vi "Run Bfr Rx - Prepend Size.vi"(7 "Data Size":i32, 8 "error in (no error)":errorcluster, 11 "Data Buffer in":u64 format="%016x") -> (0 "error out":errorcluster, 3 "Data Buffer out":u64 format="%016x")   [LabVIEW 2016, in "UDP-Custom-Device Engine.lvlib"]
uses:
  UDP-Custom-Device Engine.lvlib
  <vilib>/NI Veristand/VeriStand Data/Library/Pointer Operations/Pointer.Write (I32).vi
  <vilib>/NI Veristand/VeriStand Data/Library/VeriStand Data.lvlib
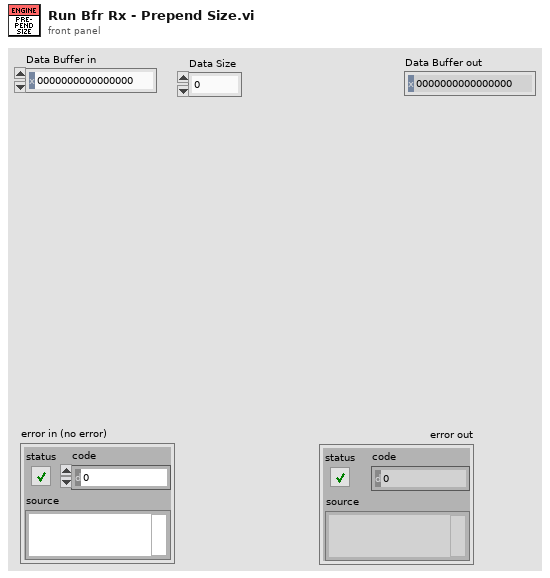
[diagram p1: front panel]
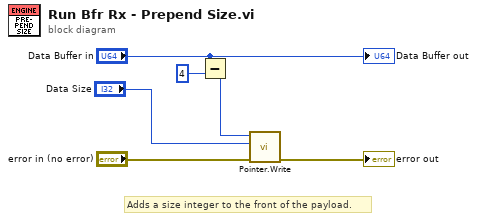
[diagram p0: block diagram]
diagram:
  # "Adds a size integer to the front of the payload."
  n1 = Subtract(x="Data Buffer in", y=u64 4) -> (x-y=w2:u64)
  n2 = call-poly <vilib>:"Pointer.Write.vi"("error in (no error)"="error in (no error)", "value"="Data Size", "pointer in"=w2) -> ("error out"=→"error out":errorcluster)  [unwired: 6 in, 2 out]
  "Data Buffer out" <- "Data Buffer in"
